vi "RTTest.vi"(9 "stop out":bool) -> ()   [LabVIEW 2022 SP3]
uses:
  <instrlib>/niScope/Controls/niScope trigger source.ctl
  <instrlib>/niScope/Configure/Trigger/niScope Configure Trigger Edge.vi
  <instrlib>/niScope/Acquire/Fetch/niScope Multi Fetch Binary 8.vi
  <vilib>/gmath/NI_Gmath.lvlib
  <vilib>/Analysis/NI_AALPro.lvlib
panel:
  out "size(s)":i32
  out "# elements in queue":i32
  out "Intensity Graph":dbl[][](graph)
  out "Fetch:Records Done":i32
  out "batches":i32
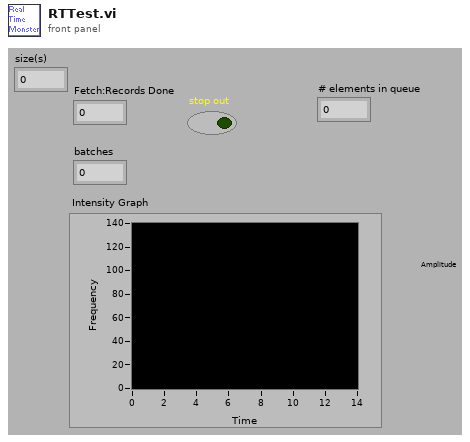
[diagram p1: front panel]
types:
  T1 = typedef "niScope trigger source.ctl" = string
  T2 = cluster{"actualSamples":i32, "absoluteInitialX":dbl, "relativeInitialX":dbl, "xIncrement":dbl, "offset":dbl, "gain":dbl, "reserved1":dbl, "reserved2":dbl}[]
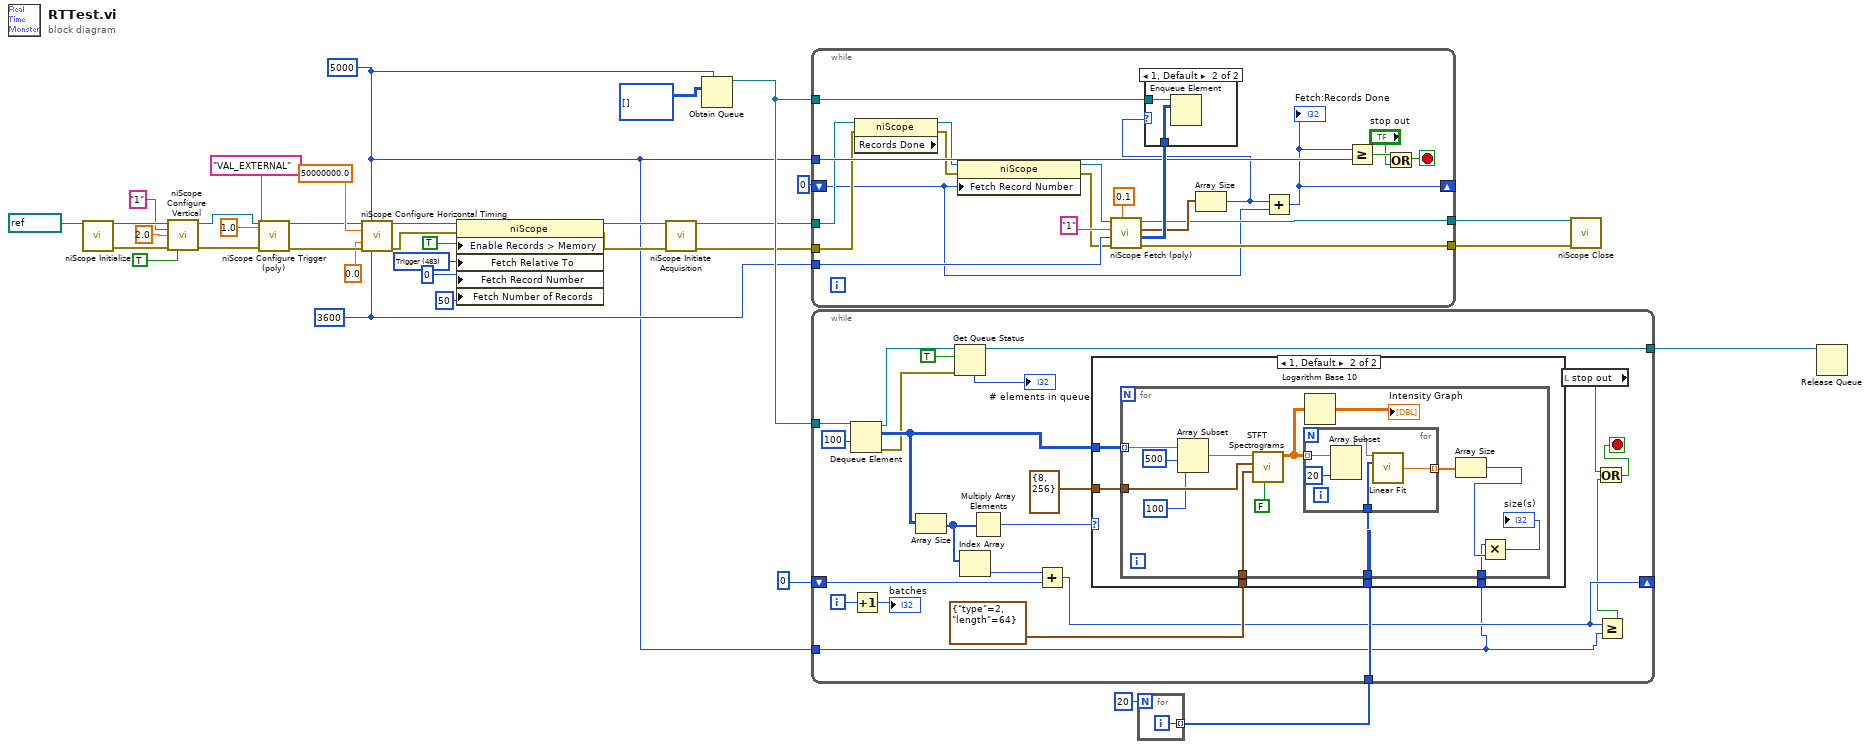
[diagram p0: block diagram]
diagram:
  w2 = 483 items=["Start"=482, "Trigger"=483, "Pretrigger"=477, "Now"=481, "Read Pointer"=388] ("Fetch:Fetch Relative To")
  w22 = 3600 ("min record length")
  w5 = 5000 ("number of records")
  n1 = call <instrlib>:"niScope Initialize.vi"("resource name"=refnum<k15> "DIG1") -> ("instrument handle"=w16:refnum<k15>, "error out"=w15:errorcluster)  [unwired: 13 in]
  n2 = call <instrlib>:"niScope Configure Vertical.vi"("instrument handle"=w16, "channels"="1", "vertical range"=2.0, "error in"=w15, "channel enabled"=TRUE) -> ("instrument handle out"=w13:refnum<k15>, "error out"=w14:errorcluster)  [unwired: 9 in]
  n3 = call-poly <instrlib>:"niScope Configure Trigger (poly).vi"("instrument handle"=w13, "trigger source"=T1 "VAL_EXTERNAL", "trigger level"=1.0, "error in"=w14) -> ("instrument handle out"=w9:refnum<k15>, "error out"=w8:errorcluster)  [unwired: 10 in]
  n4 = call <instrlib>:"niScope Configure Horizontal Timing.vi"("instrument handle"=w9, "number of records"=w5, "min sample rate"=50000000.0, "reference position"=0.0, "error in"=w8, "min record length"=w22) -> ("instrument handle out"=w29:refnum<k15>, "error out"=w26:errorcluster)  [unwired: 8 in]
  n5 = property class="niScope"(reference=w29, error in=w26, "Enable Records > Memory"=TRUE ("Horizontal:Enable Records > Memory"), "Fetch Relative To"=w2, "Fetch Record Number"=0, "Fetch Number of Records"=50) -> (reference out=w32:refnum<k15>, error out=w27:errorcluster)
  n6 = call <instrlib>:"niScope Initiate Acquisition.vi"("instrument handle"=w32, "error in"=w27) -> ("instrument handle out"=w31:refnum<k15>, "error out"=w23:errorcluster)  [unwired: 1 in, 11 out]
  n7 = Obtain Queue(max queue size (-1, unlimited)=w5, element data type=i8[][] [] ("Array")) -> (queue out=w35:refnum<queue>)  [unwired: 2 in, 3 out]
  n8 = while {
    tunnel: w35 -> [w56]
    tunnel: w31 -> [w41]
    tunnel: w23 -> [w40]
    tunnel: w22 -> [w53]
    shift-right: [w44] -> _
    shift-left: 0 -> [w39]
    tunnel: w5 -> [w50]
    tunnel: [w45] -> w4
    tunnel: [w43] -> w3
    stop <- w47 stop-if-true
    n9 = property class="niScope" props=["Records Done"](reference=w41, error in=w40) -> (reference out=w37:refnum<k15>, error out=w36:errorcluster)  [unwired: 1 out]
    n10 = property class="niScope"(reference=w37, error in=w36, "Fetch Record Number"=w39) -> (reference out=w52:refnum<k15>, error out=w38:errorcluster)
    n11 = call-poly <instrlib>:"niScope Fetch (poly).vi"("timeout"=0.1, "error in"=w38, "numSamples"=w53, "channels"="1", "instrument handle"=w52) -> ("error out"=w43:errorcluster, "wfm"=w54:i8[][], "wfm info"=w46:T2, "instrument handle out"=w45:refnum<k15>)  [unwired: 3 out]
    n12 = Array Size(array=w46) -> (size(s)=w42:i32)
    n13 = case shown="1, Default" w42 {
      tunnel: w56 -> [_ w58]
      tunnel: w54 -> [_ w57]
      frame 0 {
      }
      frame 1, Default {
        n14 = Enqueue Element(queue=w58, element=w57) -> ()  [unwired: 2 in, 3 out]
      }
    }
    n15 = Add(x=w42, y=w39) -> (x+y=w44:i32)
    "Fetch:Records Done" <- w44
    n16 = Greater Or Equal?(x=w44, y=w50) -> (x >= y?=w49:bool)
    n17 = Or(x=w49, y="stop out") -> (x .or. y?=w47:bool)
  }
  n18 = for {
    N: 20 ("dimension size") -> [_]
    tunnel: [w59] -> w19 mode=indexing
    i -> [w59]
  }
  n19 = while {
    tunnel: w35 -> [w78]
    tunnel: [w73] -> w34
    tunnel: w19 -> [w75]
    shift-right: [w64] -> _
    shift-left: 0 -> [w66]
    tunnel: w5 -> [w62]
    i -> [w81]
    stop <- w70 stop-if-true
    n20 = Dequeue Element(queue=w78, timeout in ms (-1)=100) -> (queue out=w74:refnum<queue>, element=w72:i8[][], error out=w68:errorcluster)  [unwired: 1 in, 1 out]
    n21 = Increment(x=w81) -> (x+1=→"batches":i32)
    n22 = Array Size(array=w72) -> (size(s)=w67:i32[])
    n23 = Get Queue Status(queue=w74, return elements? (F)=TRUE, error in (no error)=w68) -> (queue out=w73:refnum<queue>, # elements in queue=→"# elements in queue":i32)  [unwired: 6 out]
    n24 = Index Array(array=w67) -> (element=w65:i32)  [unwired: 1 in]
    n25 = Multiply Array Elements(1:w67) -> (0:w69:i32)
    n26 = Add(x=w65, y=w66) -> (x+y=w64:i32)
    n27 = case shown="1, Default" w69 {
      tunnel: w72 -> [_ w86]
      tunnel: cluster{"time steps":i32, "frequency bins":i32} {"time steps"=8, "frequency bins"=256} ("time-freq sampling info") -> [_ w85]
      tunnel: cluster{"type":u32, "length":i32} {"type"=2, "length"=64} ("window info") -> [_ w84]
      tunnel: w75 -> [_ w83]
      tunnel: w62 -> [_ w82]
      frame 0 {
      }
      frame 1, Default {
        n28 = for {
          tunnel: w86 -> [w96] mode=indexing
          tunnel: w85 -> [w100]
          tunnel: w84 -> [w99]
          tunnel: w83 -> [w97]
          tunnel: w82 -> [w90]
          n29 = Array Subset(array=w96, index=500, length=100) -> (w95:i8[])
          n30 = call <vilib>:"STFT Spectrograms.vi"("energy conservation?"=FALSE, "window info"=w99, "time-freq sampling info"=w100, "X"=w95) -> ("STFT Spectrogram {X}"=w88:dbl[][])  [unwired: 6 in, 1 out]
          n31 = for {
            tunnel: w88 -> [w104] mode=indexing
            tunnel: w97 -> [w105]
            tunnel: [w101] -> w92 mode=indexing
            n32 = Array Subset(array=w104, length=20) -> (w103:dbl[])  [unwired: 1 in]
            n33 = call <vilib>:"Linear Fit.vi"("Y"=w103, "X"=w105) -> ("intercept"=w101:dbl)  [unwired: 9 in, 4 out]
          }
          n34 = Logarithm Base 10(1:w88) -> (0:→"Intensity Graph":dbl[][])
          n35 = Array Size(array=w92) -> (size(s)=w91:i32)
          n36 = Multiply(x=w90, y=w91) -> (x*y=→"size(s)":i32)
        }
      }
    }
    n37 = local read "stop out"() -> (w71:bool)
    n38 = Greater Or Equal?(x=w64, y=w62) -> (x >= y?=w63:bool)
    n39 = Or(x=w71, y=w63) -> (x .or. y?=w70:bool)
  }
  n40 = call <instrlib>:"niScope Close.vi"("instrument handle"=w4, "error in"=w3) -> ()  [unwired: 13 in, 1 out]
  n41 = Release Queue(queue=w34) -> ()  [unwired: 2 in, 3 out]
